vi "verify unique parameter in range.vi"(6 "lower limit":dbl, 7 "parameter name":string, 8 "error in (no error)":errorcluster, 9 "value":dbl, 10 "upper limit":dbl, 11 "Simulated_CCD_Camera in":refnum<class "Simulated Camera.lvclass">) -> (0 "error out":errorcluster, 3 "Simulated_CCD_Camera out":refnum<class "Simulated Camera.lvclass">)   [LabVIEW 2018, in "Simulated Camera.lvclass"]
uses:
  Simulated Camera.lvclass
  <vilib>/ErrorRing/Error Ring.xnode
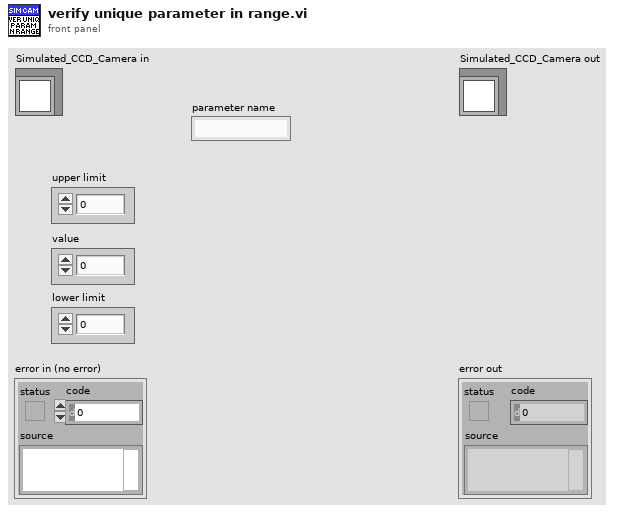
[diagram p1: front panel]
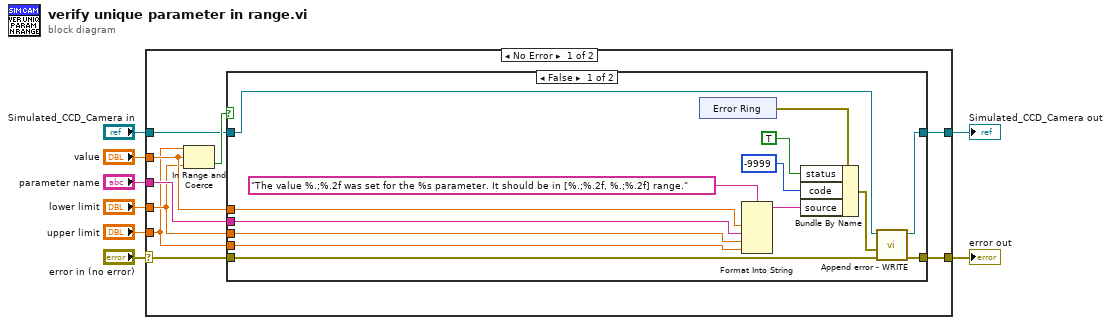
[diagram p0: block diagram]
diagram:
  n1 = case shown="No Error" "error in (no error)" {
    selector: "error in (no error)" -> [w13 w36]
    tunnel: [w12 w36] -> w7
    tunnel: [w17 w35] -> w6
    tunnel: "Simulated_CCD_Camera in" -> [w14 w35]
    tunnel: "lower limit" -> [w10 _]
    tunnel: "value" -> [w11 _]
    tunnel: "upper limit" -> [w9 _]
    tunnel: "parameter name" -> [w15 _]
    frame No Error {
      n2 = In Range and Coerce(upper limit=w9, x=w11, lower limit=w10) -> (In Range?=w16:bool)  [unwired: 1 out]
      n3 = case shown="False" w16 {
        tunnel: [w22 w34] -> w17
        tunnel: w14 -> [w21 w34]
        tunnel: w15 -> [w25 _]
        tunnel: w13 -> [w20 w33]
        tunnel: [w19 w33] -> w12
        tunnel: w11 -> [w27 _]
        tunnel: w10 -> [w24 _]
        tunnel: w9 -> [w23 _]
        frame False {
          n4 = xnode "Error Ring"() -> ("error out"=w31:errorcluster)
          n5 = Format Into String(format string="The value %.;%.2f was set for the %s parameter. It should be in [%.;%.2f, %.;%.2f] range." ("string"), w27, w25, w24, w23) -> (resulting string=w26:string)  [unwired: 2 in, 1 out]
          n6 = Bundle By Name(cluster=w31, "status"=TRUE, "code"=-9999, "source"=w26) -> (w18:errorcluster)
          n7 = call "Append error - WRITE.vi"("error in (no error)"=w20, "error"=w18, "Simulated_CCD_Camera in"=w21) -> ("error out"=w19:errorcluster, "Simulated_CCD_Camera out"=w22:refnum<class "Simulated Camera.lvclass">)  [unwired: 7 in]
        }
        frame True {
        }
      }
    }
    frame Error {
    }
  }
  "error out" <- w7
  "Simulated_CCD_Camera out" <- w6
